vi "Temperature Monitor.vi"() -> ()   [LabVIEW 2011]
doc: "This VI is the solution to an exercise in the LabVIEW Core I course.\n\nIt is used to demonstrate While loops and waveform charts. This VI takes a temperature reading from the temperature sensor on the DAQ signal accessory once every 500 ms and plots the data in a strip chart."
panel:
  out "Temperature History":dbl(graph)
  in  "Power":bool=TRUE
  # "ON\n\nOFF"
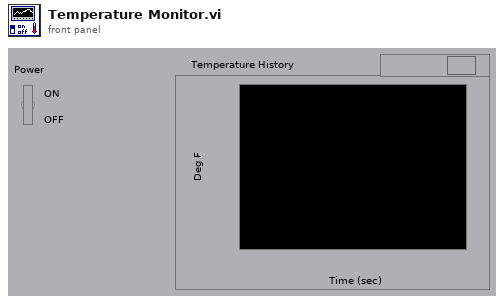
[diagram p1: front panel]
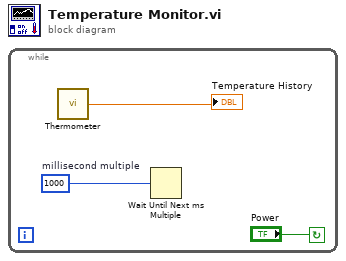
[diagram p0: block diagram]
diagram:
  n1 = while {
    stop <- "Power" continue-if-true
    w2 = u32 1000  # millisecond multiple
    n2 = call "Thermometer.vi"() -> ("Temperature"=→"Temperature History":dbl)  [unwired: 1 in]
    n3 = Wait Until Next ms Multiple(millisecond multiple=w2) -> ()  [unwired: 1 out]
  }
